vi "TeleOP Angle Val.vi"(9 "TeleOP Angle (in)":dbl, 10 "Add":bool, 11 "Write":bool) -> (1 "TeleOP Angle (out)":dbl)   [LabVIEW 2016]
uses:
  Framework/Robot Global Data.vi
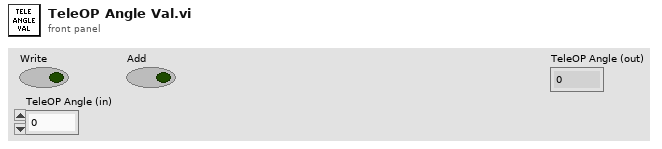
[diagram p1: front panel]
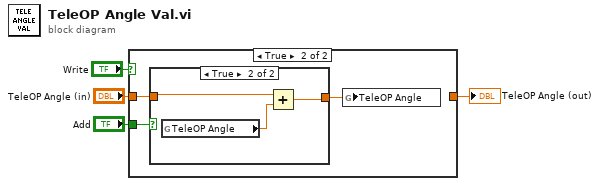
[diagram p0: block diagram]
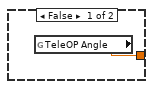
[diagram p2: hidden frame]
diagram:
  n1 = case shown="True" "Write" {
    tunnel: "TeleOP Angle (in)" -> [_ w6]
    tunnel: [w5 _] -> w2
    tunnel: "Add" -> [_ w8]
    frame False {
      n2 = global read "Robot Global Data.vi" "TeleOP Angle"() -> (w5:dbl)
    }
    frame True {
      n3 = case shown="True" w8 {
        tunnel: [w9 w11] -> w7
        tunnel: w6 -> [w9 w12]
        frame False {
        }
        frame True {
          n4 = global read "Robot Global Data.vi" "TeleOP Angle"() -> (w10:dbl)
          n5 = Add(x=w12, y=w10) -> (x+y=w11:dbl)
        }
      }
      n6 = global write "Robot Global Data.vi" "TeleOP Angle"(w7) -> ()
    }
  }
  "TeleOP Angle (out)" <- w2
